vi "Configure DC Isolation.vi"(7 "DC Isolation State (F:Disable)":bool, 8 "error in (no error)":errorcluster, 9 "DC Isolation Range (3: 20 mA)":i32(ring)=3 items=["20u", "200u", "2m", "20m", "100m"], 10 "Enable Auto Range (T:Enable)":bool=TRUE, 11 "VISA resource name":refnum<visa-resource-name>) -> (0 "error out":errorcluster, 3 "VISA resource name out":refnum<visa-resource-name>)   [LabVIEW 2017, in "Agilent E4980.lvlib"]
doc: "Configures the DC Isolation state and the range: either enables the auto range function for DC Isolation measurement, or selects specific DC Isolatioin range.\n\n<B>Notes:</B>\n(1) The DC Bias current isolation feature prevents DC current from affecting the measurement circuit.\n\n(2) If your instrument installs <B>Option 001</B> (Power and DC Bias enhancement), you can set DC Bias up to 40V. You can use IDC monitor to check the DC Bias current actually applied to the DUT."
uses:
  Agilent E4980.lvlib
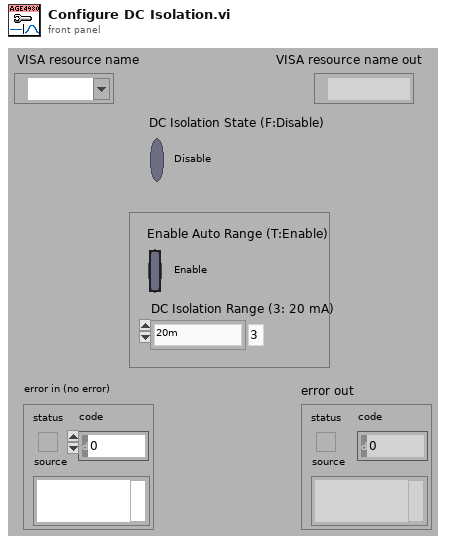
[diagram p1: front panel]
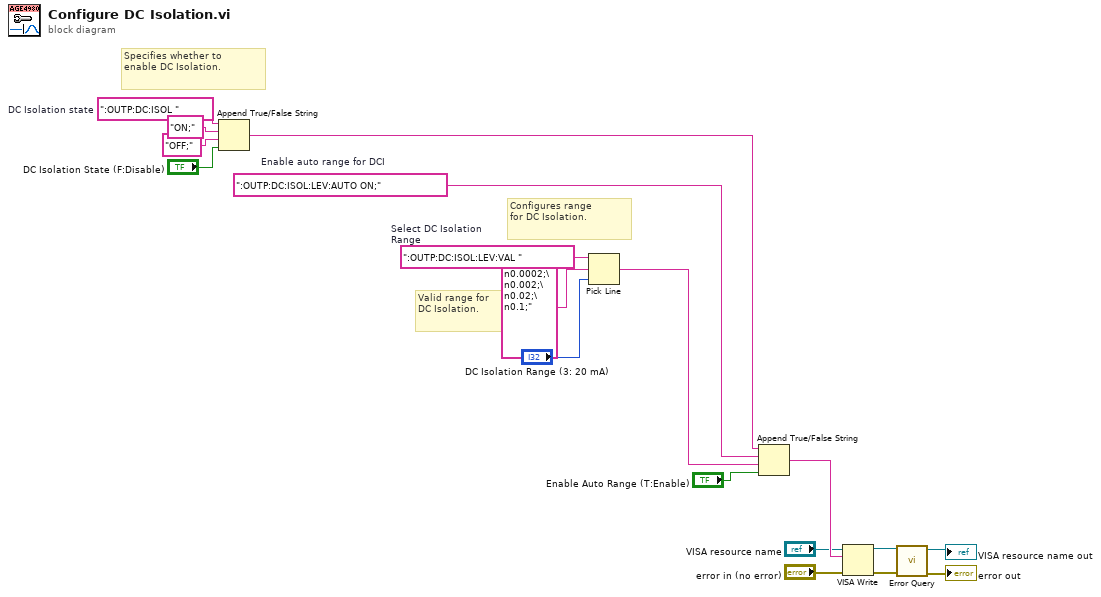
[diagram p0: block diagram]
diagram:
  w4 = ":OUTP:DC:ISOL:LEV:VAL "  # Select DC Isolation Range
  w14 = ":OUTP:DC:ISOL:LEV:AUTO ON;"  # Enable auto range for DCI
  w18 = ":OUTP:DC:ISOL "  # DC Isolation state
  # "Configures range\nfor DC Isolation."
  # "Specifies whether to\nenable DC Isolation."
  # "Valid range for\nDC Isolation."
  n1 = Append True/False String(1:"DC Isolation State (F:Disable)", 2:"OFF;" ("false string"), 3:"ON;" ("true string"), 4:w18) -> (0:w5:string)
  n2 = Pick Line(string ("")=w4, multi-line string="2E-5;\n0.0002;\n0.002;\n0.02;\n0.1;", line index="DC Isolation Range (3: 20 mA)") -> (output string=w1:string)
  n3 = Append True/False String(1:"Enable Auto Range (T:Enable)", 2:w1, 3:w14, 4:w5) -> (0:w11:string)
  n4 = VISA Write(VISA resource name="VISA resource name", write buffer=w11, error in (no error)="error in (no error)") -> (VISA resource name out=w10:refnum<visa-resource-name>, error out=w9:errorcluster)  [unwired: 1 out]
  n5 = call "Error Query.vi"("error in (no error)"=w9, "VISA resource name"=w10) -> ("error out"=→"error out":errorcluster, "VISA resource name out"=→"VISA resource name out":refnum<visa-resource-name>)  [unwired: 6 in, 2 out]
